vi "PXI-4132 Updated Channels (RT).vi"(5 "Channel Type":T1 items=["Voltage Controlled", "Current Controlled"], 7 "Channel":string, 8 "error in (no error)":errorcluster, 9 "FIFO Indexes":i32[](array[numeric]), 10 "Data In":dbl[](array[numeric]), 11 "resource name In":refnum<k15>) -> (0 "error out":errorcluster, 2 "Data Out":dbl[](array[numeric]), 3 "resource name Out":refnum<k15>)   [LabVIEW 2013, in "PXI-4132 Custom Device.lvlib"]
uses:
  PXI-4132 Custom Device.lvlib
  Channel Type.ctl
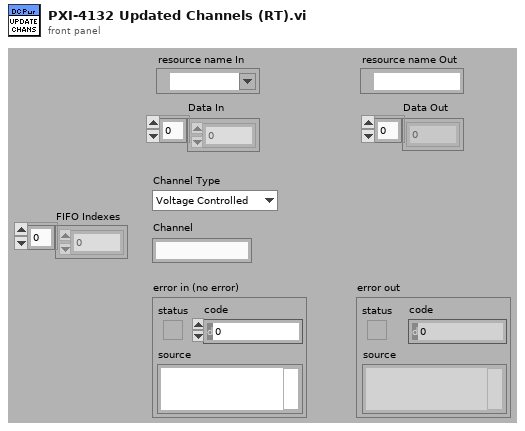
[diagram p1: front panel]
types:
  T1 = typedef "PXI-4132 Custom Device.lvlib/Channel Type.ctl" = i32
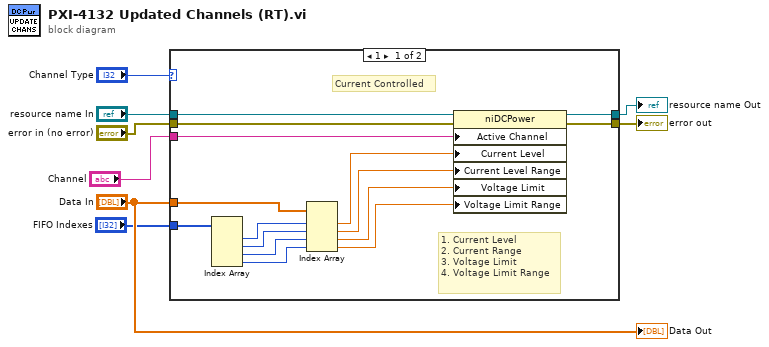
[diagram p0: block diagram]
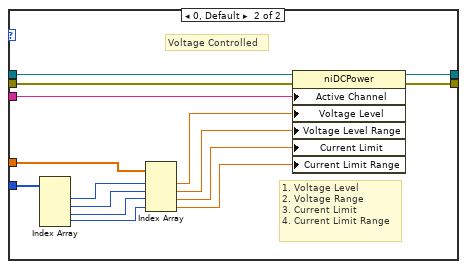
[diagram p2: hidden frame]
diagram:
  n1 = case shown="1" "Channel Type" {
    tunnel: "resource name In" -> [w23 w38]
    tunnel: "Data In" -> [w22 w37]
    tunnel: [w18 w33] -> w6
    tunnel: [w17 w32] -> w7
    tunnel: "error in (no error)" -> [w16 w31]
    tunnel: "Channel" -> [w14 w29]
    tunnel: "FIFO Indexes" -> [w13 w28]
    frame 1 {
      # "1. Current Level\n2. Current Range\n3. Voltage Limit\n4. Voltage Limit Range"
      # "Current Controlled"
      n2 = Index Array(array=w13) -> (element #1=w12:i32, element #2=w11:i32, element #3=w10:i32, element #4=w9:i32)  [unwired: 4 in]
      n3 = Index Array(array=w22, index #1=w12, index #2=w11, index #3=w10, index #4=w9) -> (element #1=w15:dbl, element #2=w21:dbl, element #3=w20:dbl, element #4=w19:dbl)
      n4 = property class="niDCPower"(reference=w23, error in=w16, "Active Channel"=w14, "Current Level"=w15, "Current Level Range"=w21, "Voltage Limit"=w20, "Voltage Limit Range"=w19) -> (reference out=w18:refnum<k15>, error out=w17:errorcluster)
    }
    frame 0, Default {
      # "1. Voltage Level\n2. Voltage Range\n3. Current Limit\n4. Current Limit Range"
      # "Voltage Controlled"
      n5 = Index Array(array=w28) -> (element #1=w27:i32, element #2=w26:i32, element #3=w25:i32, element #4=w24:i32)  [unwired: 4 in]
      n6 = Index Array(array=w37, index #1=w27, index #2=w26, index #3=w25, index #4=w24) -> (element #1=w30:dbl, element #2=w36:dbl, element #3=w35:dbl, element #4=w34:dbl)
      n7 = property class="niDCPower"(reference=w38, error in=w31, "Active Channel"=w29, "Voltage Level"=w30, "Voltage Level Range"=w36, "Current Limit"=w35, "Current Limit Range"=w34) -> (reference out=w33:refnum<k15>, error out=w32:errorcluster)
    }
  }
  "resource name Out" <- w6
  "error out" <- w7
  "Data Out" <- "Data In"
